vi "CRYSet Number Format Front Panel.vi"(11 "Vi Ref":refnum<vi>) -> ()   [LabVIEW 2013]
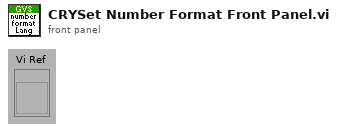
[diagram p1: front panel]
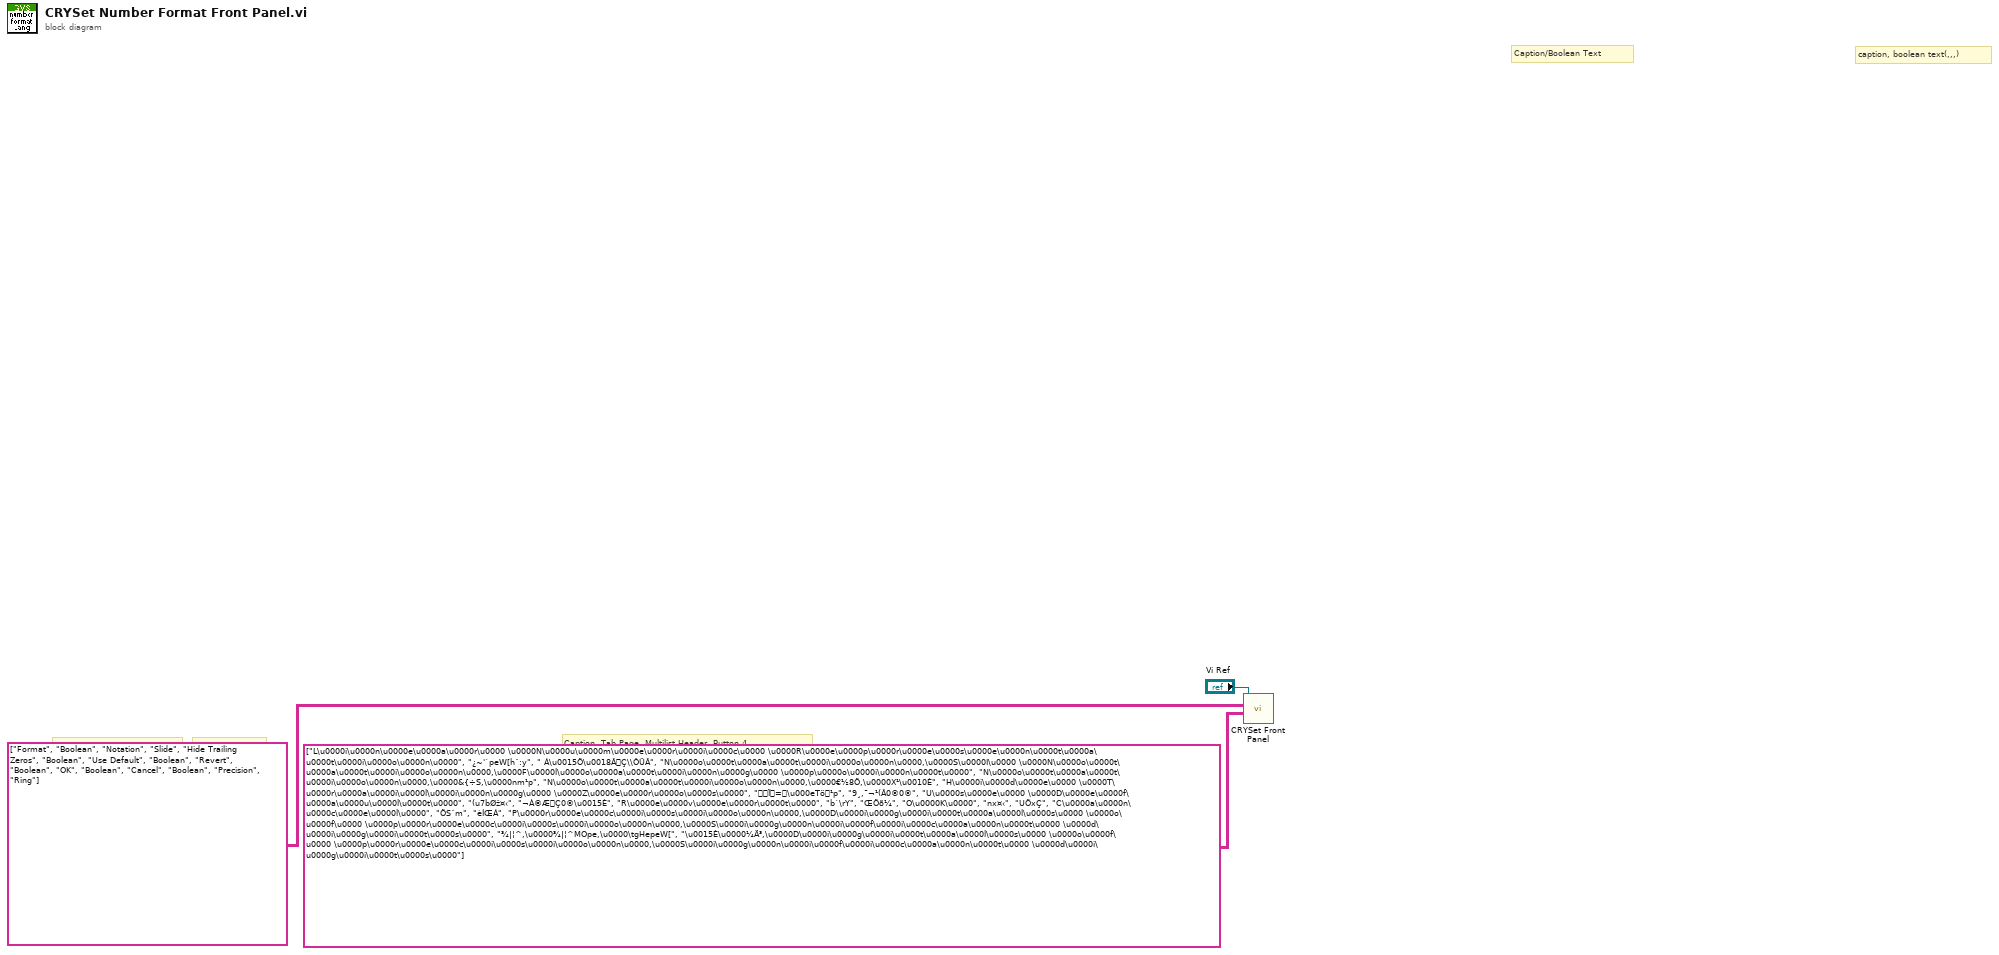
[diagram p0: block diagram]
diagram:
  # "Caption, Tab Page, Multilist Header, Button 4"
  # "Control Type"
  # "Control Name and Tab"
  # "caption, boolean text(,,,)"
  # "Caption/Boolean Text"
  n1 = call "CRYSet Front Panel.vi"("Caption(Boolean Text)"=string[][] [["L\u0000i\u0000n\u0000e\u0000a\u0000r\u0000 \u0000N\u0000u\u0000m\u0000e\u0000r\u0000i\u0000c\u0000 \u0000R\u0000e\u0000p\u0000r\u0000e\u0000s\u0000e\u0000n\u0000t\u0000a\u0000t\u0000i\u0000o\u0000n\u0000", "¿~'`peW[hˆ:y", " Á\u0015Ö\u0018ÂÇ\\ÔÜÂ"], ["N\u0000o\u0000t\u0000a\u0000t\u0000i\u0000o\u0000n\u0000,\u0000S\u0000I\u0000 \u0000N\u0000o\u0000t\u0000a\u0000t\u0000i\u0000o\u0000n\u0000,\u0000F\u0000l\u0000o\u0000a\u0000t\u0000i\u0000n\u0000g\u0000 \u0000p\u0000o\u0000i\u0000n\u0000t\u0000", "N\u0000o\u0000t\u0000a\u0000t\u0000i\u0000o\u0000n\u0000,\u0000&{÷S,\u0000nm¹p", "N\u0000o\u0000t\u0000a\u0000t\u0000i\u0000o\u0000n\u0000,\u0000€½8Ö,\u0000X¹\u0010È"], ["H\u0000i\u0000d\u0000e\u0000 \u0000T\u0000r\u0000a\u0000i\u0000l\u0000i\u0000n\u0000g\u0000 \u0000Z\u0000e\u0000r\u0000o\u0000s\u0000", "Ï=\u000eTö¹p", "9¸,¯¬¹(Â0®0®"], ["U\u0000s\u0000e\u0000 \u0000D\u0000e\u0000f\u0000a\u0000u\u0000l\u0000t\u0000", "(u7bØž¤‹", "¬À©ÆÇ0®\u0015È"], ["R\u0000e\u0000v\u0000e\u0000r\u0000t\u0000", "b`\rY", "ŒÖõ¼"], ["O\u0000K\u0000", "nx¤‹", "UÖxÇ"], ["C\u0000a\u0000n\u0000c\u0000e\u0000l\u0000", "ÖSˆm", "èÍŒÁ"], ["P\u0000r\u0000e\u0000c\u0000i\u0000s\u0000i\u0000o\u0000n\u0000,\u0000D\u0000i\u0000g\u0000i\u0000t\u0000a\u0000l\u0000s\u0000 \u0000o\u0000f\u0000 \u0000p\u0000r\u0000e\u0000c\u0000i\u0000s\u0000i\u0000o\u0000n\u0000,\u0000S\u0000i\u0000g\u0000n\u0000i\u0000f\u0000i\u0000c\u0000a\u0000n\u0000t\u0000 \u0000d\u0000i\u0000g\u0000i\u0000t\u0000s\u0000", "¾|¦^,\u0000¾|¦^MOpe,\u0000\tgHepeW[", "\u0015È\u0000¼Ä³,\u0000D\u0000i\u0000g\u0000i\u0000t\u0000a\u0000l\u0000s\u0000 \u0000o\u0000f\u0000 \u0000p\u0000r\u0000e\u0000c\u0000i\u0000s\u0000i\u0000o\u0000n\u0000,\u0000S\u0000i\u0000g\u0000n\u0000i\u0000f\u0000i\u0000c\u0000a\u0000n\u0000t\u0000 \u0000d\u0000i\u0000g\u0000i\u0000t\u0000s\u0000"]], "Control ID and Type(Label Name, Type)"=string[][] [["Format", "Boolean"], ["Notation", "Slide"], ["Hide Trailing Zeros", "Boolean"], ["Use Default", "Boolean"], ["Revert", "Boolean"], ["OK", "Boolean"], ["Cancel", "Boolean"], ["Precision", "Ring"]], "Vi Ref"="Vi Ref") -> ()  [unwired: 9 in]
